vi "SendLine.vi"(8 "error in (no error)":errorcluster caption="Fehler (Eingang, kein Fehler)", 10 "SendString":string, 11 "MoveoSerial Eingang":refnum<class "MoveoSerial.lvclass">) -> (0 "error out":errorcluster caption="Fehler (Ausgang)", 3 "MoveoSerial Ausgang":refnum<class "MoveoSerial.lvclass">)   [LabVIEW 2019, in "MoveoSerial.lvclass"]
uses:
  MoveoSerial.lvclass
  MoveoSerial.lvclass/MoveoSerial.ctl
panel:
  out "Verknüpfter String":string
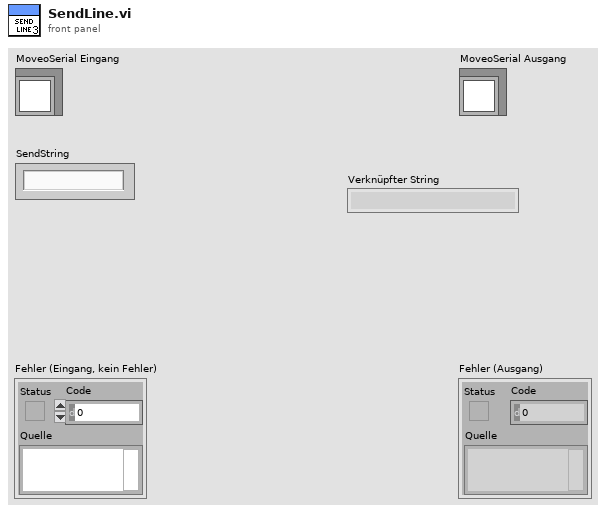
[diagram p1: front panel]
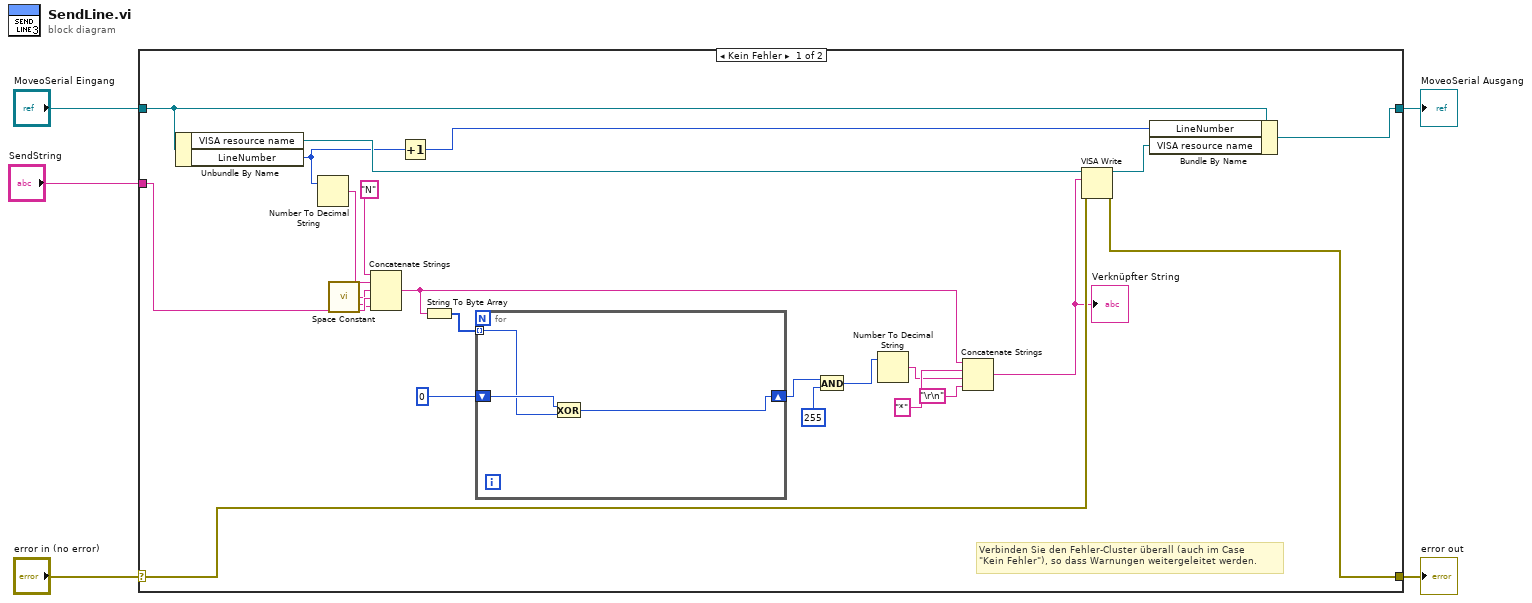
[diagram p0: block diagram]
diagram:
  n1 = case shown="Kein Fehler" "error in (no error)" {
    selector: "error in (no error)" -> [w23 w32]
    tunnel: [w22 w32] -> w4
    tunnel: [w25 w31] -> w2
    tunnel: "MoveoSerial Eingang" -> [w26 w31]
    tunnel: "SendString" -> [w20 _]
    frame No Error {
      # "Verbinden Sie den Fehler-Cluster überall (auch im Case\n\"Kein Fehler\"), so dass Warnungen weitergeleitet werden."
      n2 = Unbundle By Name(w26) -> ("VISA resource name"=w27:refnum<visa-resource-name>, "LineNumber"=w19:u64)
      n3 = Number To Decimal String(number=w19) -> (decimal integer string=w17:string)  [unwired: 1 in]
      n4 = call <vilib>:"Space Constant.vi"() -> ("String"=w7:string)
      n5 = Concatenate Strings("N", w17, w7, w20, w7) -> (w6:string)
      n6 = Increment(x=w19) -> (x+1=w18:u64)
      n7 = String To Byte Array(string=w6) -> (unsigned byte array=w12:u8[])
      n8 = for {
        tunnel: w12 -> [w28] mode=indexing
        shift-right: [w30] -> w10
        shift-left: u8 0 -> [w29]
        n9 = Exclusive Or(1:w28, 2:w29) -> (0:w30:u8)
      }
      n10 = And(x=w10, y=u8 255) -> (x .and. y?=w9:u8)
      n11 = Number To Decimal String(number=w9) -> (decimal integer string=w15:string)  [unwired: 1 in]
      n12 = Concatenate Strings(w6, "*", w15, "\r\n") -> (w13:string)
      "Verknüpfter String" <- w13
      n13 = VISA Write(VISA resource name=w27, write buffer=w13, error in (no error)=w23) -> (VISA resource name out=w24:refnum<visa-resource-name>, error out=w22:errorcluster)  [unwired: 1 out]
      n14 = Bundle By Name(cluster=w26, "LineNumber"=w18, "VISA resource name"=w24) -> (w25:refnum<class "MoveoSerial.lvclass">)
    }
    frame Error {
    }
  }
  "error out" <- w4
  "MoveoSerial Ausgang" <- w2
